vi "Data Unsubscribed.vi"(8 "error in (no error)":errorcluster, 10 "Groups":string[](array[string]), 11 "SubscribedDataHandler in":refnum<class "SubscribedDataHandler.lvclass">) -> (0 "error out":errorcluster, 3 "SubscribedDataHandler out":refnum<class "SubscribedDataHandler.lvclass">)   [LabVIEW 2020, in "Vecto.lvlib" / "SubscribedDataHandler.lvclass"]
uses:
  SubscribedDataHandler.lvclass
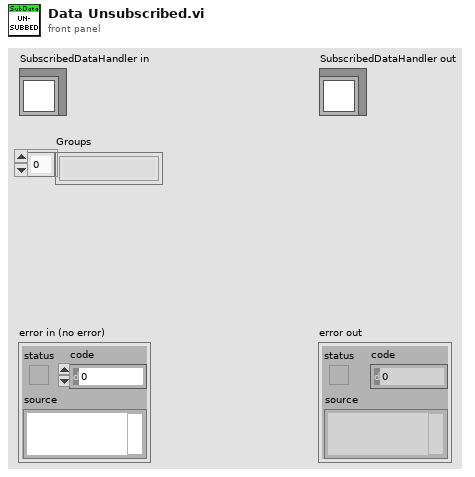
[diagram p1: front panel]
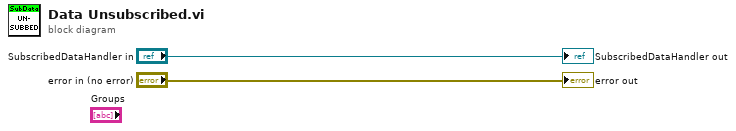
[diagram p0: block diagram]
diagram:
  "error out" <- "error in (no error)"
  "SubscribedDataHandler out" <- "SubscribedDataHandler in"
